vi "Robot_mode_notifier.vi"   [LabVIEW 2017, in "labview-standard-library.lvlib" / "universial-typedefs.lvlib"]
uses:
  <vilib>/Rock Robotics/WPI/DriverStation/WPI_DriverStationRobotMode2.ctl
  universial-typedefs.lvlib
types:
  T1 = typedef "WPI_DriverStationRobotMode2.ctl" = enum16{"Autonomous Disabled", "Autonomous Enabled", "Teleop Disabled", "Teleop Enabled", "Disconnected", "Finish", "Test Disabled", "Test Enabled", "Emergency Stopped"}
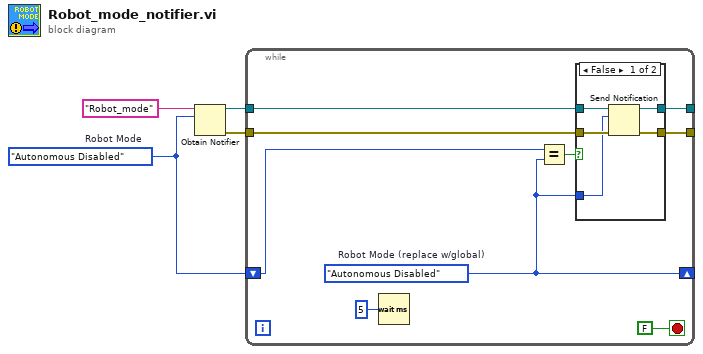
[diagram p0: block diagram]
diagram:
  w1 = WPI_DriverStationRobotMode2."Autonomous Disabled"  # Robot Mode
  n1 = Obtain Notifier(name (unnamed)="Robot_mode", notification data type=w1) -> (notifier out=w3:refnum<notifier>, error out=w2:errorcluster)  [unwired: 2 in, 1 out]
  n2 = while {
    tunnel: w3 -> [w12]
    tunnel: w2 -> [w9]
    shift-right: [w6] -> _
    shift-left: w1 -> [w7]
    tunnel: [w11] -> _
    tunnel: [w10] -> _
    stop <- FALSE stop-if-true
    w6 = WPI_DriverStationRobotMode2."Autonomous Disabled"  # Robot Mode (replace w/global)
    n3 = Wait (ms)(milliseconds to wait=u32 5) -> ()  [unwired: 1 out]
    n4 = Equal?(x=w7, y=w6) -> (x = y?=w8:bool)
    n5 = case shown="False" w8 {
      tunnel: w12 -> [w18 w19]
      tunnel: [w17 w19] -> w11
      tunnel: [w16 w20] -> w10
      tunnel: w9 -> [w15 w20]
      tunnel: w6 -> [w14 _]
      frame False {
        n6 = Send Notification(notification=w14, notifier=w18, error in (no error)=w15) -> (notifier out=w17:refnum<notifier>, error out=w16:errorcluster)
      }
      frame True {
      }
    }
  }
